vi "Change2dTo1dArray.vi"(1 "AI2去噪后数据":dbl[][](array[numeric])) -> (0 "AI2一维数组":dbl[](array[numeric]))   [LabVIEW 2018]
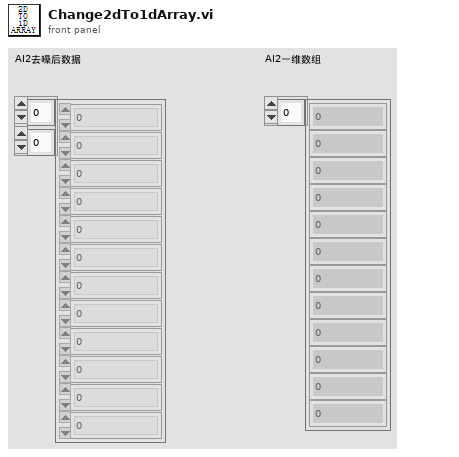
[diagram p1: front panel]
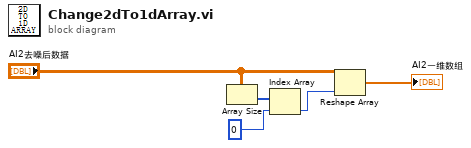
[diagram p0: block diagram]
diagram:
  n1 = Array Size(array="AI2去噪后数据") -> (size(s)=w2:i32[])
  n2 = Index Array(array=w2, index=0) -> (element=w3:i32)
  n3 = Reshape Array("AI2去噪后数据", w3) -> (→"AI2一维数组":dbl[])
